vi "set tag writer or reader.vi"(7 "module GUID":string, 8 "error in":errorcluster, 9 "channel":refnum<class "TBM channel.lvclass">, 10 "tag descriptor":refnum<class "tag descriptor.lvclass">, 11 "engine configuration in":refnum<class "engine configuration.lvclass">) -> (0 "error out":errorcluster, 3 "engine configuration out":refnum<class "engine configuration.lvclass">)   [LabVIEW 2013, in "engine configuration.lvclass"]
uses:
  engine configuration.lvclass
  <vilib>/NI/Tag Bus/tag/tag descriptor.lvclass
  <vilib>/NI/Tag Bus Module Framework/channel/TBM channel.lvclass
  engine configuration.lvclass/engine configuration.ctl
  <vilib>/NI/Tag Bus/tag/tag descriptor.lvclass/tag descriptor.ctl
  <vilib>/NI/Tag Bus Module Framework/channel/TBM channel.lvclass/TBM channel.ctl
  <vilib>/NI/Tag Bus/tag/read tag name.vi
  <vilib>/NI/Tag Bus Module Framework/channel/Read channel classification.vi
  <vilib>/NI/Tag Bus Module Framework/root configuration/TBM configuration.lvclass
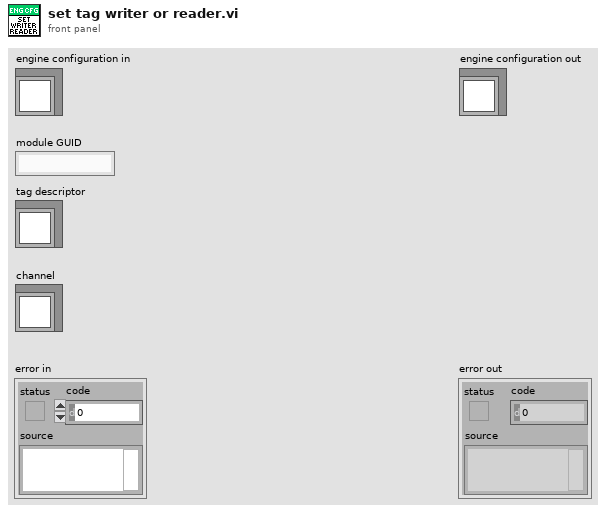
[diagram p1: front panel]
types:
  T1 = typedef "engine configuration.lvclass/Tag Info.ctl" = cluster{"Tag":refnum<class "tag descriptor.lvclass">, "Writer":string, "Readers":string[], "Owning ID":string}
  T2 = typedef "TBM channel.lvclass/channel classification.ctl" = enum16{"input data", "output data", "processing parameter", "processing result"}
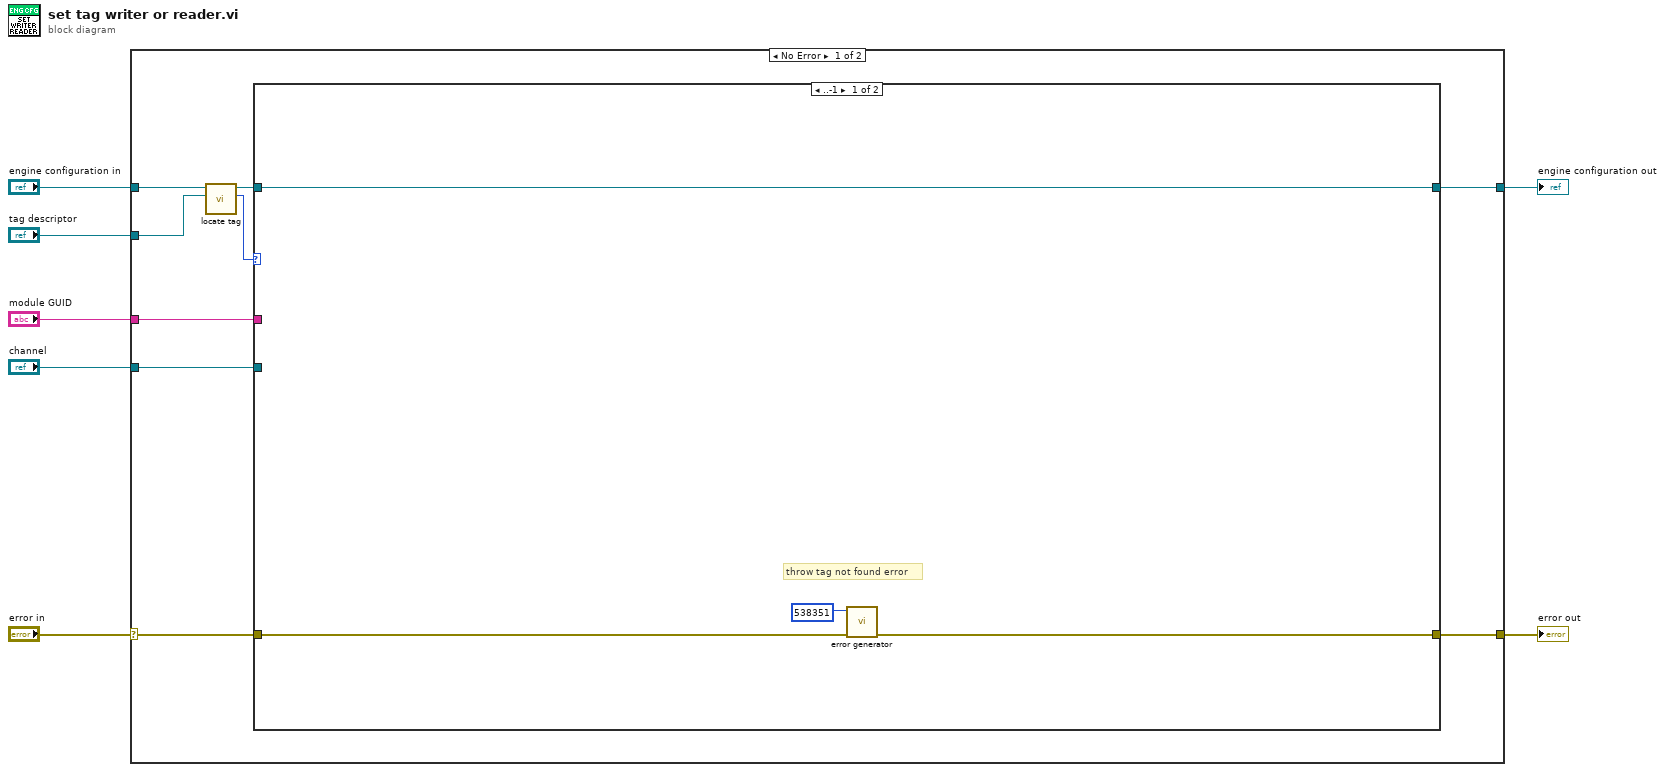
[diagram p0: block diagram]
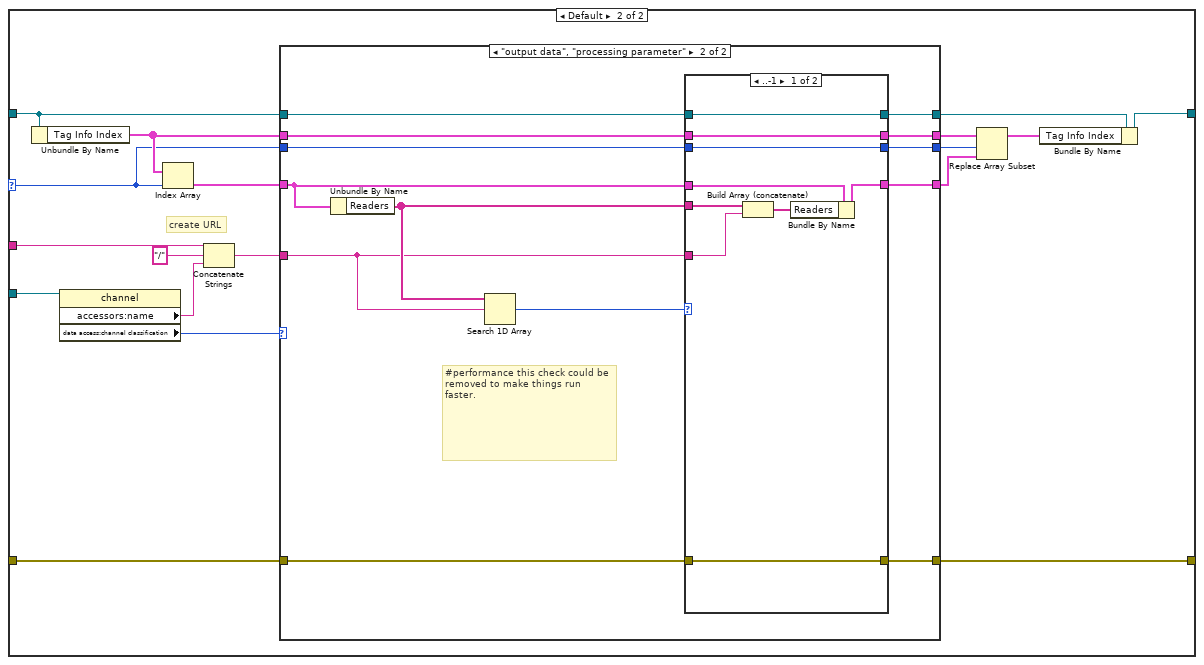
[diagram p2: hidden frame]
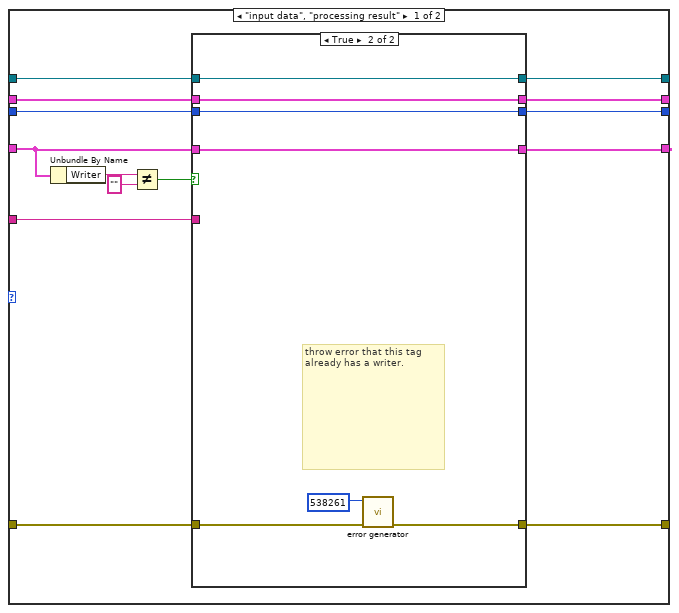
[diagram p3: hidden frame]
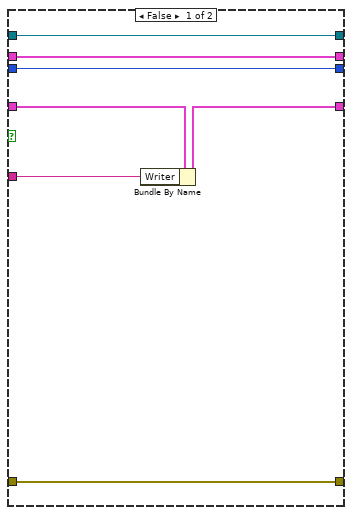
[diagram p4: hidden frame]
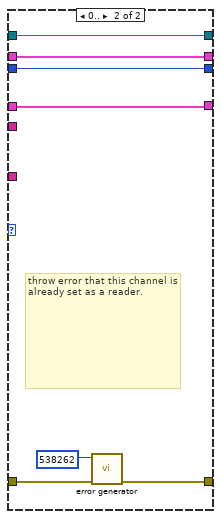
[diagram p5: hidden frame]
diagram:
  n1 = case shown="No Error" "error in" {
    selector: "error in" -> [w11 w97]
    tunnel: [w9 w97] -> w6
    tunnel: [w8 w96] -> w4
    tunnel: "engine configuration in" -> [w16 w96]
    tunnel: "tag descriptor" -> [w15 _]
    tunnel: "module GUID" -> [w12 _]
    tunnel: "channel" -> [w13 _]
    frame No Error {
      n2 = call "locate tag.vi"("tag descriptor"=w15, "engine configuration in"=w16) -> ("index"=w10:i32, "engine configuration out"=w14:refnum<class "engine configuration.lvclass">)  [unwired: 8 in]
      n3 = case shown="..-1" w10 {
        selector: w10 -> [_ w29]
        tunnel: w14 -> [w20 w28]
        tunnel: w13 -> [_ w38]
        tunnel: w12 -> [_ w36]
        tunnel: w11 -> [w18 w31]
        tunnel: [w17 w27] -> w9
        tunnel: [w20 w21] -> w8
        frame ..-1 {
          # "throw tag not found error"
          n4 = call <vilib>:"error generator.vi"("error in"=w18, "error code (0)"=538351) -> ("error out"=w17:errorcluster)  [unwired: 9 in]
        }
        frame Default {
          # "create URL"
          n5 = Unbundle By Name(w28) -> ("Tag Info Index"=w30:T1[])
          n6 = property class="channel"(reference=w38) -> ("accessors:name"=w35:string, "data access:channel classification"=w34:T2)  [unwired: 1 in, 2 out]
          n7 = Index Array(array=w30, index=w29) -> (element=w32:T1)
          n8 = Concatenate Strings(w36, "/" ("string"), w35) -> (w33:string)
          n9 = case shown="\"output data\", \"processing parameter\"" w34 {
            tunnel: w33 -> [w47 w68]
            tunnel: w32 -> [w48 w79]
            tunnel: w31 -> [w49 w75]
            tunnel: w30 -> [w42 w72]
            tunnel: w29 -> [w40 w70]
            tunnel: w28 -> [w45 w78]
            tunnel: [w44 w77] -> w23
            tunnel: [w46 w76] -> w24
            tunnel: [w43 w74] -> w27
            tunnel: [w41 w73] -> w25
            tunnel: [w39 w71] -> w26
            frame "input data", "processing result" {
              n10 = Unbundle By Name(w48) -> ("Writer"=w52:string)
              n11 = Not Equal?(x=w52, y="") -> (x != y?=w50:bool)
              n12 = case shown="True" w50 {
                tunnel: w49 -> [w56 w61]
                tunnel: w48 -> [w59 w66]
                tunnel: w47 -> [w58 _]
                tunnel: [w57 w66] -> w46
                tunnel: [w56 w60] -> w43
                tunnel: w45 -> [w55 w65]
                tunnel: [w55 w65] -> w44
                tunnel: w42 -> [w54 w64]
                tunnel: [w54 w64] -> w41
                tunnel: w40 -> [w53 w63]
                tunnel: [w53 w63] -> w39
                frame False {
                  n13 = Bundle By Name(cluster=w59, "Writer"=w58) -> (w57:T1)
                }
                frame True {
                  # "throw error that this tag already has a writer."
                  n14 = call <vilib>:"error generator.vi"("error in"=w61, "error code (0)"=538261) -> ("error out"=w60:errorcluster)  [unwired: 9 in]
                }
              }
            }
            frame "output data", "processing parameter" {
              # "#performance this check could be removed to make things run faster."
              n15 = Unbundle By Name(w79) -> ("Readers"=w69:string[])
              n16 = Search 1D Array(1D array=w69, element=w68) -> (index of element=w67:i32)  [unwired: 1 in]
              n17 = case shown="..-1" w67 {
                tunnel: w69 -> [w88 _]
                tunnel: w68 -> [w87 _]
                tunnel: w79 -> [w86 w94]
                tunnel: w78 -> [w84 w95]
                tunnel: [w84 w95] -> w77
                tunnel: [w83 w94] -> w76
                tunnel: w75 -> [w82 w90]
                tunnel: [w82 w89] -> w74
                tunnel: [w81 w93] -> w73
                tunnel: w72 -> [w81 w93]
                tunnel: [w80 w92] -> w71
                tunnel: w70 -> [w80 w92]
                frame ..-1 {
                  n18 = Build Array (concatenate)(w88, w87) -> (w85:string[])
                  n19 = Bundle By Name(cluster=w86, "Readers"=w85) -> (w83:T1)
                }
                frame 0.. {
                  # "throw error that this channel is already set as a reader."
                  n20 = call <vilib>:"error generator.vi"("error in"=w90, "error code (0)"=538262) -> ("error out"=w89:errorcluster)  [unwired: 9 in]
                }
              }
            }
          }
          n21 = Replace Array Subset(array=w25, new element=w24, index=w26) -> (w22:T1[])
          n22 = Bundle By Name(cluster=w23, "Tag Info Index"=w22) -> (w21:refnum<class "engine configuration.lvclass">)
        }
      }
    }
    frame Error {
    }
  }
  "error out" <- w6
  "engine configuration out" <- w4
